vi "PH_Tektronix_7000.set Channel GUI Element.vi"(2 "GUI Ref Channel":refnum<vi>, 3 "Channel Config":T1={"Enable Channel"=FALSE, "Bandwidth"=0, "Input Impedance"=0, "Vertical Coupling"=0, "Probe Attenuation"=1.0, "Range [V/div]"=1.0, "Position [div]"=10.0, "Bandwidth raw"=""} {"Vertical Coupling" items=["AC", "DC", "Ground"]; "Input Impedance" items=["1M", "50"]; "Bandwidth" items=["FULL", "500 MHz", "250 MHz", "150 MHz", "20 MHz"]}, 4 "enabled?":bool, 5 "error in":errorcluster) -> (19 "error out":errorcluster)   [LabVIEW 2014, in "PH_Tektronix_7000.lvlib"]
doc: "If the reference is valid, the incoming data are set to the GUI."
uses:
  PH_Tektronix_7000.lvlib
  PH_Tektronix_7000.Channel Config.ctl
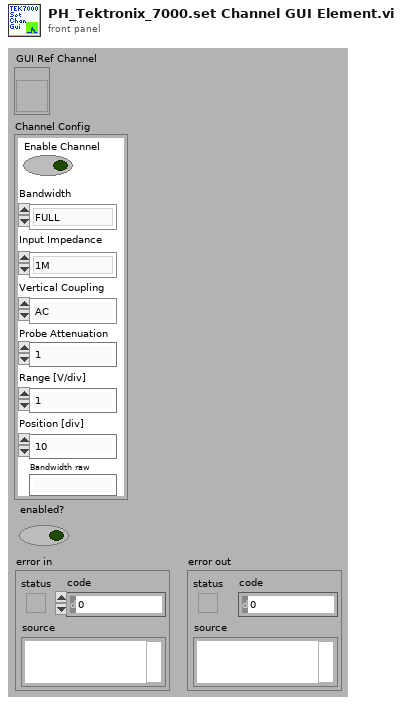
[diagram p1: front panel]
types:
  T1 = typedef "PH_Tektronix_7000.lvlib/PH_Tektronix_7000.Channel Config.ctl" = cluster{"Enable Channel":bool, "Bandwidth":u16, "Input Impedance":u16, "Vertical Coupling":u16, "Probe Attenuation":dbl, "Range [V/div]":dbl, "Position [div]":dbl, "Bandwidth raw":string}
  T2 = enum8{"Enabled", "Disabled", "Disabled and Grayed Out"}
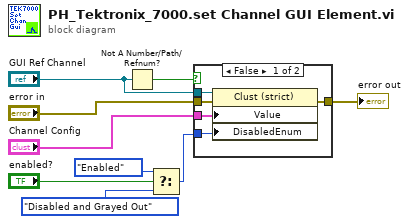
[diagram p0: block diagram]
diagram:
  n1 = Not A Number/Path/Refnum?(number/path/refnum="GUI Ref Channel") -> (NaN/Path/Refnum?=w7:bool)
  n2 = Select(t=T2."Enabled" ("Disabled"), s="enabled?", f=T2."Disabled and Grayed Out") -> (s? t:f=w3:T2)
  n3 = case shown="False" w7 {
    tunnel: "error in" -> [w14 w15]
    tunnel: [w13 w15] -> w8
    tunnel: "GUI Ref Channel" -> [w12 _]
    tunnel: "Channel Config" -> [w11 _]
    tunnel: w3 -> [w10 _]
    frame False {
      n4 = property class="Clust (strict)"(reference=w12, error in=w14, "Value"=w11, "DisabledEnum"=w10) -> (error out=w13:errorcluster)  [unwired: 1 out]
    }
    frame True {
    }
  }
  "error out" <- w8
